vi "Get G06 Stream.vi"(9 "Duration (sec)":dbl, 10 "DateTimeS":string, 11 "base path":path) -> (0 "error out":errorcluster, 3 "FileName":string)   [LabVIEW 2014]
uses:
  H264 NAL unit.ctl
panel:
  out "Rec Time":dbl
  out "Frame Count":u64
  in  "stop":bool
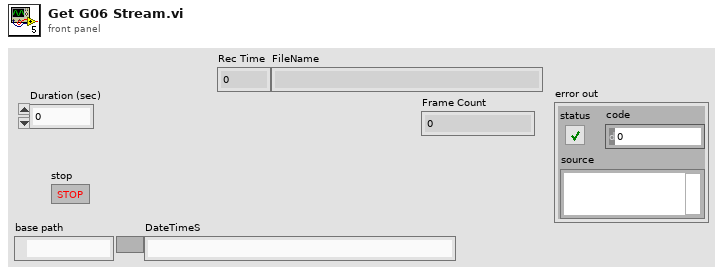
[diagram p1: front panel]
types:
  T1 = typedef "H264 NAL unit.ctl" = cluster{"forbidden_zero_bit":string, "nal_ref_idc":string, "NAL Unit type":string, "Start bit":bool, "End bit":bool, "Data":string}
  T2 = typedef "RTSP Session.ctl" = cluster{"connection ID":refnum<k5>, "Authorization (Basic)":string, "Detailed Stream":string, "DESCRIBE":string, "SETUP":string, "PLAY":string, "TEARDOWN":string}
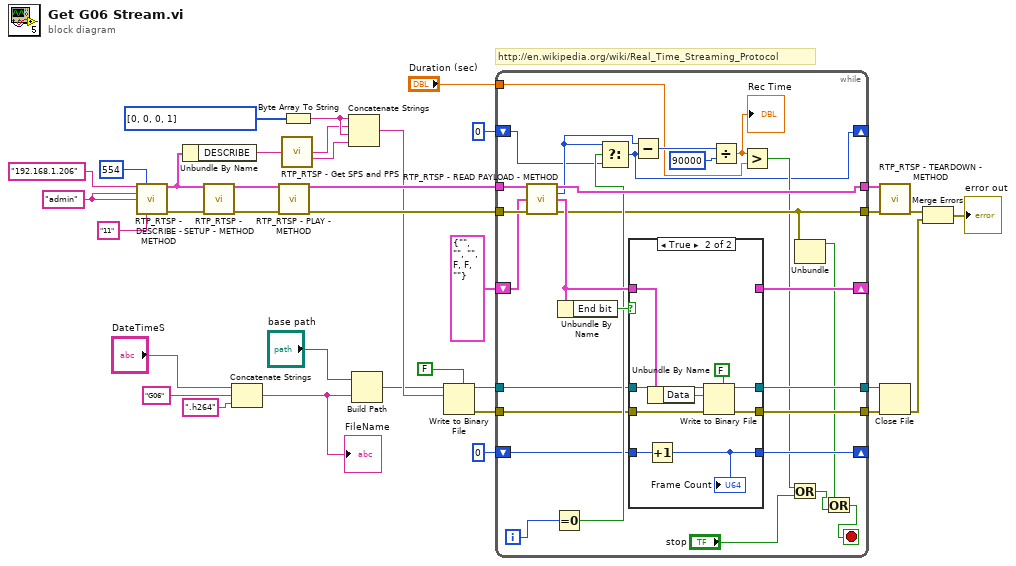
[diagram p0: block diagram]
diagram:
  w14 = "admin" ("uid")
  # "http://en.wikipedia.org/wiki/Real_Time_Streaming_Protocol"
  n1 = call "RTP_RTSP - DESCRIBE - METHOD.vi"("address"="192.168.1.206", "port"=u16 554, "uid"=w14, "pwd"=w14, "Stream File"="11") -> ("RTSP Session"=w27:T2, "error out"=w36:errorcluster)  [unwired: 9 in]
  n2 = Unbundle By Name(w27) -> ("DESCRIBE"=w26:string)
  n3 = call "RTP_RTSP - SETUP - METHOD.vi"("RTSP Session"=w27, "error in (no error)"=w36) -> ("RTSP Session 2"=w33:T2, "error out"=w34:errorcluster)  [unwired: 12 in]
  n4 = Concatenate Strings("DateTimeS", "G06" ("string"), ".h264" ("string")) -> (w10:string)
  "FileName" <- w10
  n5 = call "RTP_RTSP - PLAY - METHOD.vi"("RTSP Session"=w33, "error in (no error)"=w34) -> ("RTSP Session 2"=w32:T2, "error out"=w31:errorcluster)  [unwired: 12 in]
  n6 = call "RTP_RTSP - Get SPS and PPS.vi"("DESCRIBE"=w26) -> ("SPS"=w23:string, "PPS"=w22:string)  [unwired: 13 in]
  n7 = Byte Array To String(unsigned byte array=u8[] [0, 0, 0, 1]) -> (string=w25:string)
  n8 = Concatenate Strings(w25, w23, w25, w22) -> (w21:string)
  n9 = Build Path(base path="base path", name or relative path=w10) -> (appended path=w11:path)
  n10 = Write to Binary File(file (use dialog)=w11, data=w21, 5:FALSE ("prepend array or string size? (T)")) -> (refnum out=w19:refnum<file>, error out=w16:errorcluster)  [unwired: 3 in, 1 out]
  n11 = while {
    tunnel: w32 -> [w64]
    tunnel: w31 -> [w63]
    tunnel: [w62] -> w30
    tunnel: [w44] -> w29
    shift-right: [w58] -> _
    shift-left: T1 {"forbidden_zero_bit"="", "nal_ref_idc"="", "NAL Unit type"="", "Start bit"=FALSE, "End bit"=FALSE, "Data"=""} ("H264 NAL unit 2") -> [w61]
    shift-right: [w37] -> _
    shift-left: u32 0 ("timestamp") -> [w52]
    tunnel: w19 -> [w51]
    tunnel: [w50] -> w18
    tunnel: [w49] -> w17
    tunnel: w16 -> [w48]
    shift-right: [w46] -> _
    shift-left: u64 0 -> [w47]
    tunnel: "Duration (sec)" -> [w38]
    i -> [w55]
    stop <- w45 stop-if-true
    n12 = call "RTP_RTSP - READ PAYLOAD - METHOD.vi"("RTSP Session"=w64, "H264 NAL unit"=w61, "error in (no error)"=w63) -> ("RTSP Session 2"=w62:T2, "timestamp"=w53:u32, "H264 NAL unit 2"=w59:T1, "error out"=w44:errorcluster)  [unwired: 9 in]
    n13 = Equal To 0?(x=w55) -> (x = 0?=w54:bool)
    n14 = Unbundle By Name(w59) -> ("End bit"=w60:bool)
    n15 = Select(t=w53, s=w54, f=w52) -> (s? t:f=w37:u32)
    n16 = case shown="True" w60 {
      tunnel: w59 -> [w68 w72]
      tunnel: [w68 _] -> w58
      tunnel: w51 -> [w67 w77]
      tunnel: [w67 w76] -> w50
      tunnel: [w66 w74] -> w49
      tunnel: w48 -> [w66 w75]
      tunnel: [w65 w69] -> w46
      tunnel: w47 -> [w65 w70]
      frame False {
      }
      frame True {
        n17 = Increment(x=w70) -> (x+1=w69:u64)
        "Frame Count" <- w69
        n18 = Unbundle By Name(w72) -> ("Data"=w71:string)
        n19 = Write to Binary File(file (use dialog)=w77, data=w71, error in=w75, 5:FALSE ("prepend array or string size? (T)")) -> (refnum out=w76:refnum<file>, error out=w74:errorcluster)  [unwired: 2 in, 1 out]
      }
    }
    n20 = Subtract(x=w53, y=w37) -> (x-y=w57:u32)
    n21 = Divide(x=w57, y=u32 90000) -> (x/y=w39:dbl)
    "Rec Time" <- w39
    n22 = Greater?(x=w39, y=w38) -> (0:w40:bool)
    n23 = Or(x=w40, y="stop") -> (x .or. y?=w41:bool)
    n24 = Unbundle(w44) -> ("status"=w43:bool)  [unwired: 2 out]
    n25 = Or(x=w43, y=w41) -> (x .or. y?=w45:bool)
  }
  n26 = call "RTP_RTSP - TEARDOWN - METHOD.vi"("RTSP Session"=w30, "error in (no error)"=w29) -> ("error out"=w6:errorcluster)  [unwired: 12 in, 1 out]
  n27 = Close File(refnum=w18, error in=w17) -> (error out=w5:errorcluster)  [unwired: 1 out]
  n28 = Merge Errors(w6, w5) -> (→"error out":errorcluster)
